vi "Clear-68016.vi"(1 "error in (no error)":errorcluster) -> (0 "error out":errorcluster)   [LabVIEW 2020]
doc: "This VI is to clear the error -2532 when opening a VI which saved in LabVIEW's old versions."
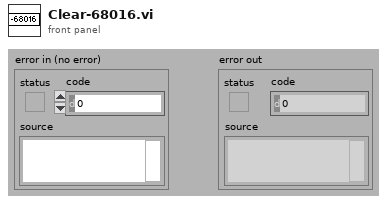
[diagram p1: front panel]
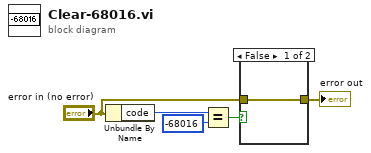
[diagram p0: block diagram]
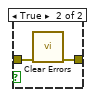
[diagram p2: hidden frame]
diagram:
  n1 = Unbundle By Name("error in (no error)") -> ("code"=w3:i32)
  n2 = Equal?(x=w3, y=-68016) -> (x = y?=w1:bool)
  n3 = case shown="False" w1 {
    tunnel: [w6 w8] -> w5
    tunnel: "error in (no error)" -> [w6 w7]
    frame False {
    }
    frame True {
      n4 = call <vilib>:"Clear Errors.vi"("error in (no error)"=w7) -> ("error out"=w8:errorcluster)  [unwired: 1 in, 5 out]
    }
  }
  "error out" <- w5
